vi "EjectDisc.vi"() -> ()   [LabVIEW 2018]
uses:
  <vilib>/Rock Robotics/WPI/Solenoid/WPI_SolenoidValue.ctl
  <vilib>/Rock Robotics/WPI/Solenoid/WPI_SolenoidSetEnum.vi
panel:
  in  "Disc Eject":bool
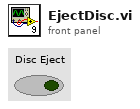
[diagram p1: front panel]
types:
  T1 = typedef "WPI_SolenoidValue.ctl" = enum16{"Off", "On", "Forward", "Reverse"}
  T2 = typedef "WPI_SolenoidDevRef.ctl" = cluster{"DevStatus":errorcluster, "Pneumatics Control Module":u8, "Forward Solenoid Channel":T3, "Reverse Solenoid Channel":T3}
  T3 = typedef "WPI_SolenoidChannel.ctl" = enum8{"Solenoid 0", "Solenoid 1", "Solenoid 2", "Solenoid 3", "Solenoid 4", "Solenoid 5", "Solenoid 6", "Solenoid 7", "Invalid"}
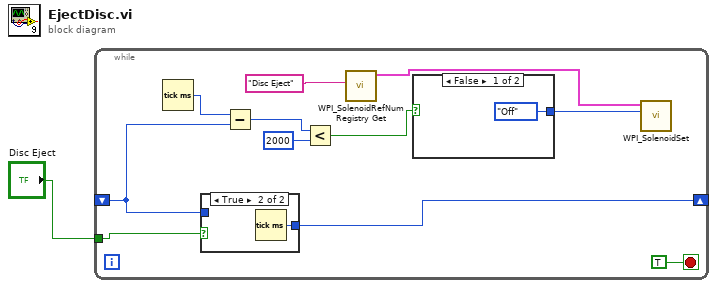
[diagram p0: block diagram]
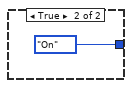
[diagram p2: hidden frame]
diagram:
  n1 = while {
    tunnel: "Disc Eject" -> [w12]
    shift-right: [w11] -> _
    shift-left: _ -> [w6]
    stop <- TRUE stop-if-true
    n2 = Tick Count (ms)() -> (millisecond timer value=w10:u32)
    n3 = case shown="True" w12 {
      tunnel: [w15 w16] -> w11
      tunnel: w6 -> [w15 _]
      frame False {
      }
      frame True {
        n4 = Tick Count (ms)() -> (millisecond timer value=w16:u32)
      }
    }
    n5 = Subtract(x=w10, y=w6) -> (x-y=w9:u32)
    n6 = Less?(x=w9, y=u32 2000) -> (x < y?=w8:bool)
    n7 = call <vilib>:"WPI_SolenoidRefNum Registry Get.vi"("refnum name"="Disc Eject") -> ("SolenoidDevRef"=w4:T2)  [unwired: 9 in, 1 out]
    n8 = case shown="False" w8 {
      tunnel: [WPI_SolenoidValue."Off" ("Value") WPI_SolenoidValue."On" ("Value")] -> w3
      frame False {
      }
      frame True {
      }
    }
    n9 = call-poly <vilib>:"WPI_SolenoidSet.vi"("Value"=w3, "SolenoidDevRef"=w4) -> ()  [unwired: 8 in, 2 out]
  }
